vi "读取配置.vi"() -> (3 "输入簇":T1)   [LabVIEW 2016, in "数据查询.lvlib"]
uses:
  <vilib>/Utility/config.llb/NI_LVConfig.lvlib
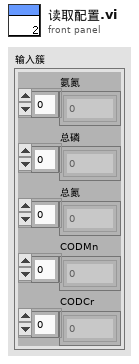
[diagram p1: front panel]
types:
  T1 = cluster{"氨氮":dbl[], "总磷":dbl[], "总氮":dbl[], "CODMn":dbl[], "CODCr":dbl[]}
  T2 = typedef "NI_LVConfig.lvlib/Config Data RefNum.ctl" = refnum<k1>
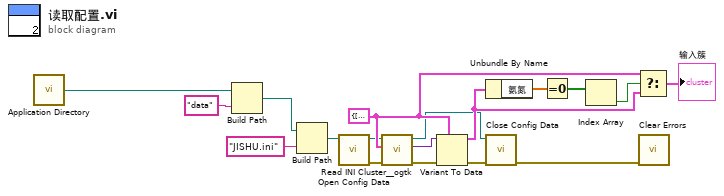
[diagram p0: block diagram]
diagram:
  w15 = T1 {"氨氮"=[0.2, 0.05, 0.1, 0.1], "总磷"=[0.02, 0.05, 0.1, 0.1], "总氮"=[0.3, 0.05, 0.1, 0.1], "CODMn"=[1.5, 0.1, 0.1, 0.1], "CODCr"=[5.0, 0.05, 0.1, 0.1]} ("输入簇")
  n1 = call <vilib>:"Application Directory.vi"() -> ("Application Directory"=w8:path)
  n2 = Build Path(base path=w8, name or relative path="data" ("名称或相对路径")) -> (appended path=w5:path)
  n3 = Build Path(base path=w5, name or relative path="JISHU.ini" ("名称或相对路径")) -> (appended path=w7:path)
  n4 = call <vilib>:"Open Config Data.vi"("configuration file path"=w7) -> ("error out"=w10:errorcluster, "refnum"=w9:T2)  [unwired: 8 in, 1 out]
  n5 = call <userlib>:"Read INI Cluster__ogtk.vi"("error in (no error)"=w10, "INI Fomatted Cluster Type"=w15, "refnum"=w9) -> ("error out"=w13:errorcluster, "INI Fomatted Cluster"=w12:variant, "dup refnum"=w11:T2)  [unwired: 4 in, 2 out]
  n6 = Variant To Data(error in=w13, type=w15, Variant=w12) -> (data=w16:T1, error out=w14:errorcluster)
  n7 = Unbundle By Name(w16) -> ("氨氮"=w17:dbl[])
  n8 = call <vilib>:"Close Config Data.vi"("error in (no error)"=w14, "refnum"=w11) -> ("error out"=w1:errorcluster)  [unwired: 8 in, 1 out]
  n9 = Equal To 0?(x=w17) -> (x = 0?=w2:bool[])
  n10 = Index Array(array=w2) -> (element=w3:bool)  [unwired: 1 in]
  n11 = Select(t=w15, s=w3, f=w16) -> (s? t:f=→"输入簇":T1)
  n12 = call <vilib>:"Clear Errors.vi"("error in (no error)"=w1) -> ()  [unwired: 5 in, 2 out]
